vi "moving_average.vi"(0 "y":dbl format="%.2f") -> ()   [LabVIEW 2016]
doc: "Moving average,\n\nThis program calculates and displays the moving average, with a pre-selected number. First of all, the program initialized two shift registers. The top shift register is initialized with one element and this register continiously adds the previous value with the new value. This shift register keeps the total of the last xx measurements. When dividing the results of the add function with the pre-selected value, we can calculate the moving average value. The bottom shift register contains an array with the dimension \"Average\". This shift register keeps all values of the measurement. The replacement function replaces every loop the new value. \n \nThis method is very efficent and fast, because we using the replace element function inside the loop and before we enter the while loop we initialzes the array. This VI was created in LabVIEW 6.1."
panel:
  in  "stop":bool
  out "?":cluster{dbl, dbl}(graph)
  in  "Average":i32=25
  # "Select the moving average and then\nrun the VI.  The chart will show the\ncurrent measurement and the \nresulting moving average."
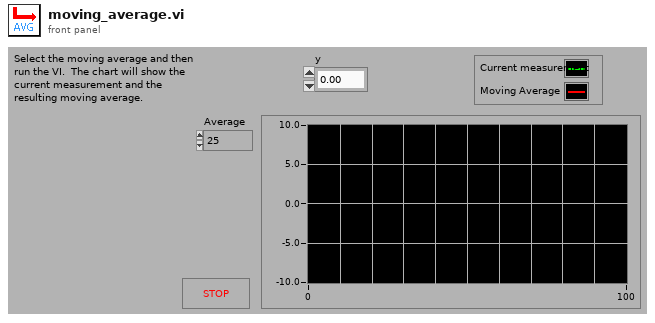
[diagram p1: front panel]
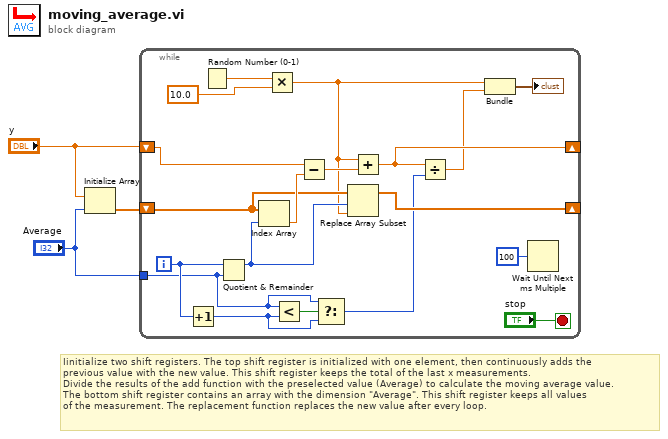
[diagram p0: block diagram]
diagram:
  # "Iinitialize two shift registers. The top shift register is initialized with one element, then continuously adds the \nprevious value with the new value. This shift register keeps the total of the last x measurements. \nDivide the results of the add function with the preselected value (Average) to calculate the moving average value.\nThe bottom shift register contains an array with the dimension \"Average\". This shift register keeps all values \nof the measurement. The replacement function replaces the new value after every loop."
  n1 = Initialize Array("y", "Average") -> (w3:dbl[])
  n2 = while {
    tunnel: "Average" -> [w4]
    shift-left: w3 -> [w19]
    shift-right: [w21] -> _
    shift-left: "y" -> [w17]
    shift-right: [w15] -> _
    i -> [w10]
    stop <- "stop" stop-if-true
    n3 = Increment(x=w10) -> (x+1=w7:i32)
    n4 = Random Number (0-1)() -> (number: 0 to 1=w6:dbl)
    n5 = Quotient & Remainder(x=w10, y=w4) -> (x-y*floor(x/y)=w16:i32)  [unwired: 1 out]
    n6 = Index Array(array=w19, index=w16) -> (element=w20:dbl)
    n7 = Multiply(x=w6, y=10.0) -> (x*y=w14:dbl)
    n8 = Less?(x=w4, y=w7) -> (x < y?=w9:bool)
    n9 = Subtract(x=w17, y=w20) -> (x-y=w18:dbl)
    n10 = Select(t=w4, s=w9, f=w7) -> (s? t:f=w8:i32)
    n11 = Replace Array Subset(array=w19, new element=w14, index=w16) -> (w21:dbl[])
    n12 = Add(x=w14, y=w18) -> (x+y=w15:dbl)
    n13 = Divide(x=w15, y=w8) -> (x/y=w13:dbl)
    n14 = Bundle(w14, w13) -> (→"?":cluster{dbl, dbl})  [unwired: 1 in]
    n15 = Wait Until Next ms Multiple(millisecond multiple=u32 100) -> ()  [unwired: 1 out]
  }
